vi "TimeCal.vi"(9 "Speed In":dbl format="%#_13g", 10 "Command":string, 11 "controller in":refnum<k24>) -> (2 "Time(ms)":dbl, 3 "controller out":refnum<k24>)   [LabVIEW 2016]
uses:
  C:/Users/TTUHEP/Documents/LabVIEW/Other Models/2010/Bin/Aerotech.A3200.dll
  Other Models/2010/Bin/Aerotech.A3200.dll
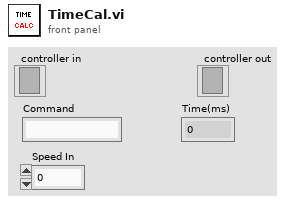
[diagram p1: front panel]
types:
  T1 = typedef "ControllerDiagPacket.ctl" = cluster{"Number of Diag Packets":i32, "Axes":T2[], "error":errorcluster}
  T2 = typedef "AxisDiagPacket.ctl" = cluster{"Axis Name":string, "Analog Input 0":dbl, "Analog Input 1":dbl, "Axis Fault (num)":i32, "Axis Fault (str)":string, "Axis Fault (bits)":cluster{"AmplifierFault":bool, "AmplifierTemperatureFault":bool, "CcwEndOfTravelLimitFault":bool, "CcwSoftwareLimitFault":bool, "CommunicationLostFault":bool, "CwEndOfTravelLimitFault":bool, "CwSoftwareLimitFault":bool, "EmergencyStopFault":bool, "EncoderFault":bool, "ExternalFault":bool, "FeedbackScalingFault":bool, "GantryMisalignFault ":bool, "HallSensorFault":bool, "InPositionTimeoutFault":bool, "InternalFault":bool, "MarkerSearchFault":bool, "MaxVelocityCommandFault":bool, "MissedInterruptFault":bool, "MotorTemperatureFault":bool, "None":bool, "OverCurrentFault":bool, "PositionErrorFault":bool, "PositionFeedbackFault":bool, "PowerSupplyFault":bool, "ProbeInputFault":bool, "SafeZoneFault":bool, "VelocityErrorFault":bool, "VelocityFeedbackFault":bool, "VoltageClampFault":bool}, "Axis Status (num)":i32, "Axis Status (str)":string, "Axis Status (bits)":cluster{"BacklashActive":bool, "CalibrationEnabled1D":bool, "CalibrationEnabled2D":bool, "CommandValid":bool, "DriveAbortPending":bool, "DrivePending":bool, "Enabling":bool, "GainMappingEnabled":bool, "GantryAligned":bool, "GantryRealigning":bool, "Homed":bool, "Homing":bool, "IFOVEnabled":bool, "JogGenerating":bool, "Jogging":bool, "JoystickControl":bool, "MasterSlaveControl":bool, "MotionBlocked":bool, "MotionClamped":bool, "MoveDone":bool, "None":bool, "NotVirtual":bool, "Profiling":bool, "Stability0":bool, "Stability1":bool, "TrajectoryFiltering":bool, "WaitDone":bool}, "Current Command":sgl, "Current Error":sgl, "Current Feedback":sgl, "Digital Inputs":i32, "Digital Outputs":i32, "Drive Status":i32, "Drive Status (str)":string, "Drive Status (bits)":cluster{"AccelerationPhase":bool, "AutofocusActive":bool, "BrakeOutput":bool, "CcwEndOfTravelLimitInput":bool, "CosineEncoderError":bool, "CurrentClamp":bool, "CwEndOfTravelLimitInput":bool, "DecelerationPhase":bool, "DualLoopActive":bool, "EmergencyStopInput":bool, "Enabled":bool, "EncoderClipping":bool, "GalvoCalibrationEnabled":bool, "GalvoPowerCorrection":bool, "HallAInput":bool, "HallBInput":bool, "HallCInput":bool, "HighResolutionMode":bool, "HomeLimitInput":bool, "InPosition":bool, "InPosition2":bool, "MarkerInput":bool, "MarkerLatch":bool, "MoveActive":bool, "NoMotorSupply":bool, "None":bool, "PowerLimiting":bool, "ProgrammingFlash":bool, "ProgrammingMXH":bool, "PSOHaltLatch":bool, "ServoControl":bool, "SineEncoderError":bool}, "Position Feedback Auxiliary":dbl, "Position Command":dbl, "Position Error":dbl, "Position Feedback":dbl, "Program Position Command":dbl, "Program Position Error":dbl, "Program Position Feedback":dbl, "Velocity Command":dbl, "Velocity Error":dbl, "Velocity Feedback":dbl}
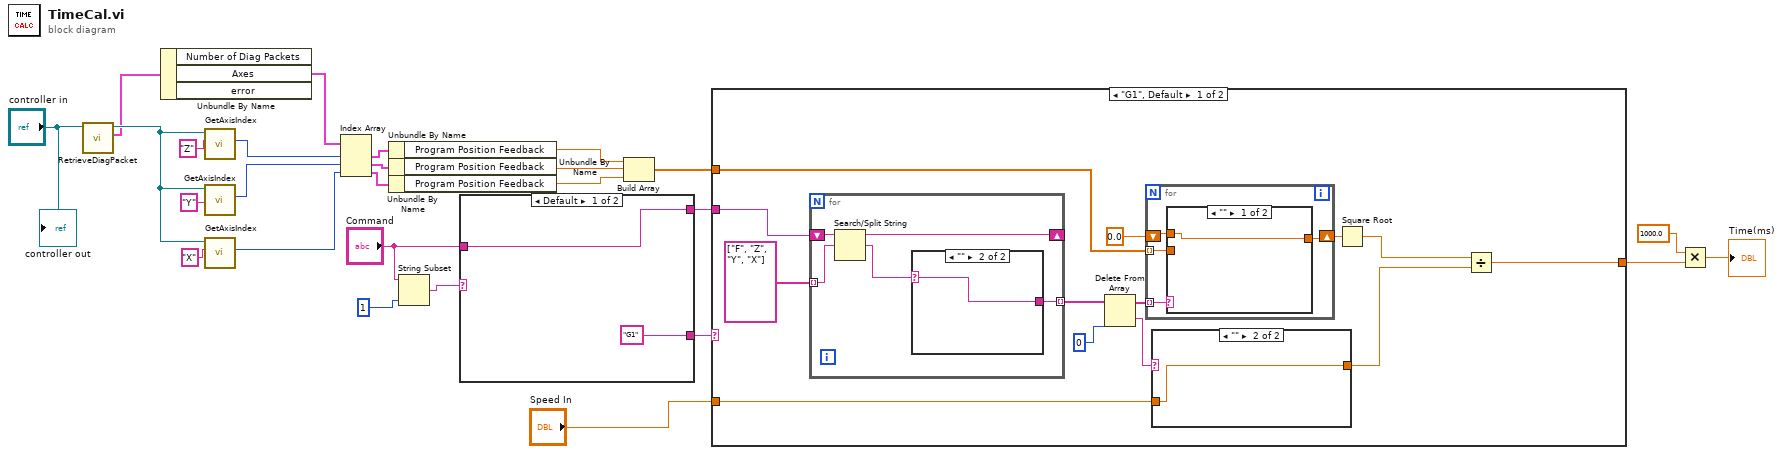
[diagram p0: block diagram]
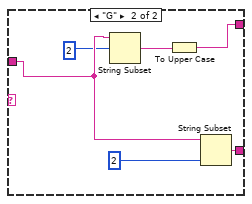
[diagram p2: hidden frame]
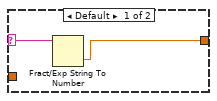
[diagram p3: hidden frame]
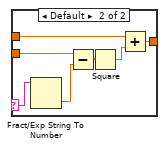
[diagram p4: hidden frame]
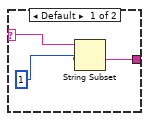
[diagram p5: hidden frame]
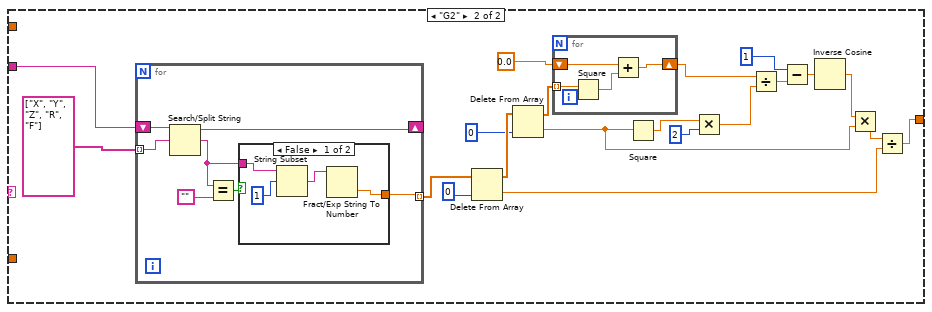
[diagram p6: hidden frame]
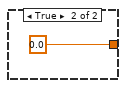
[diagram p7: hidden frame]
diagram:
  n1 = call "RetrieveDiagPacket.vi"("Controller In"="controller in") -> ("ControllerDiagPacket"=w16:T1, "Controller Out"=w20:refnum<k24>)  [unwired: 8 in, 1 out]
  n2 = Unbundle By Name(w16) -> ("Axes"=w15:T2[])  [unwired: 2 out]
  n3 = call "GetAxisIndex.vi"("axis name"="Z", "controller in"=w20) -> ("axis index"=w14:i32)  [unwired: 7 in, 2 out]
  n4 = call "GetAxisIndex.vi"("axis name"="Y", "controller in"=w20) -> ("axis index"=w13:i32)  [unwired: 7 in, 2 out]
  n5 = call "GetAxisIndex.vi"("axis name"="X", "controller in"=w20) -> ("axis index"=w12:i32)  [unwired: 7 in, 2 out]
  n6 = Index Array(array=w15, index #1=w14, index #2=w13, index #3=w12) -> (element #1=w11:T2, element #2=w10:T2, element #3=w9:T2)
  n7 = Unbundle By Name(w11) -> ("Program Position Feedback"=w8:dbl)
  n8 = Unbundle By Name(w10) -> ("Program Position Feedback"=w7:dbl)
  n9 = Unbundle By Name(w9) -> ("Program Position Feedback"=w6:dbl)
  n10 = String Subset(string="Command", length (rest)=1) -> (substring=w2:string)  [unwired: 1 in]
  n11 = case shown="Default" w2 {
    tunnel: ["G1" w34] -> w26
    tunnel: [w27 w33] -> w25
    tunnel: "Command" -> [w27 w30]
    frame Default {
    }
    frame "G" {
      n12 = String Subset(string=w30, offset (0)=2) -> (substring=w31:string)  [unwired: 1 in]
      n13 = To Upper Case(1:w31) -> (0:w33:string)
      n14 = String Subset(string=w30, length (rest)=2) -> (substring=w34:string)  [unwired: 1 in]
    }
  }
  n15 = Build Array(w8, w7, w6) -> (w5:dbl[])
  n16 = case shown="\"G1\", Default" w26 {
    tunnel: w25 -> [w46 w90]
    tunnel: [w39 w72] -> w24
    tunnel: w5 -> [w38 _]
    tunnel: "Speed In" -> [w36 _]
    frame "G1", Default {
      n17 = for {
        tunnel: string[] ["F", "Z", "Y", "X"] -> [w67] mode=indexing
        shift-right: [w65] -> _
        shift-left: w46 -> [w66]
        tunnel: [w64] -> w45 mode=indexing
        n18 = Search/Split String(string=w66, search string/char (-)=w67) -> (substring before match=w65:string, match + rest of string=w63:string)  [unwired: 1 in, 1 out]
        n19 = case shown="\"\"" w63 {
          selector: w63 -> [w68 w71]
          tunnel: [w69 w71] -> w64
          frame Default {
            n20 = String Subset(string=w68, offset (0)=1) -> (substring=w69:string)  [unwired: 1 in]
          }
          frame "" {
          }
        }
      }
      n21 = Delete From Array(array=w45, index=0) -> (deleted portion=w37:string, array with subset deleted=w43:string[])  [unwired: 1 in]
      n22 = for {
        tunnel: w43 -> [w53] mode=indexing
        shift-right: [w54] -> w41
        shift-left: 0.0 -> [w52]
        tunnel: w38 -> [w51] mode=indexing
        n23 = case shown="\"\"" w53 {
          selector: w53 -> [_ w57]
          tunnel: [w55 w61] -> w54
          tunnel: w52 -> [w55 w59]
          tunnel: w51 -> [_ w58]
          frame "" {
          }
          frame Default {
            n24 = Fract/Exp String To Number(string=w57) -> (number=w56:dbl)  [unwired: 3 in, 1 out]
            n25 = Subtract(x=w58, y=w56) -> (x-y=w60:dbl)
            n26 = Square(x=w60) -> (x^2=w62:dbl)
            n27 = Add(x=w59, y=w62) -> (x+y=w61:dbl)
          }
        }
      }
      n28 = case shown="\"\"" w37 {
        selector: w37 -> [w49 _]
        tunnel: w36 -> [_ w50]
        tunnel: [w48 w50] -> w35
        frame Default {
          n29 = Fract/Exp String To Number(string=w49) -> (number=w48:dbl)  [unwired: 3 in, 1 out]
        }
        frame "" {
        }
      }
      n30 = Square Root(x=w41) -> (sqrt(x)=w40:dbl)
      n31 = Divide(x=w40, y=w35) -> (x/y=w39:dbl)
    }
    frame "G2" {
      n32 = for {
        tunnel: string[] ["X", "Y", "Z", "R", "F"] -> [w101] mode=indexing
        shift-right: [w100] -> _
        shift-left: w90 -> [w102]
        tunnel: [w96] -> w89 mode=indexing
        n33 = Search/Split String(string=w102, search string/char (-)=w101) -> (substring before match=w100:string, match + rest of string=w97:string)  [unwired: 1 in, 1 out]
        n34 = Equal?(x=w97, y="") -> (x = y?=w99:bool)
        n35 = case shown="False" w99 {
          tunnel: w97 -> [w106 _]
          tunnel: [w104 0.0] -> w96
          frame False {
            n36 = String Subset(string=w106, offset (0)=1) -> (substring=w103:string)  [unwired: 1 in]
            n37 = Fract/Exp String To Number(string=w103) -> (number=w104:dbl)  [unwired: 3 in, 1 out]
          }
          frame True {
          }
        }
      }
      n38 = Delete From Array(array=w89, index=0) -> (deleted portion=w73:dbl, array with subset deleted=w87:dbl[])  [unwired: 1 in]
      n39 = Delete From Array(array=w87, index=0) -> (deleted portion=w76:dbl, array with subset deleted=w85:dbl[])  [unwired: 1 in]
      n40 = for {
        tunnel: w85 -> [w95] mode=indexing
        shift-right: [w94] -> w83
        shift-left: 0.0 -> [w93]
        n41 = Square(x=w95) -> (x^2=w92:dbl)
        n42 = Add(x=w93, y=w92) -> (x+y=w94:dbl)
      }
      n43 = Square(x=w76) -> (x^2=w82:dbl)
      n44 = Multiply(x=w82, y=2) -> (x*y=w80:dbl)
      n45 = Divide(x=w83, y=w80) -> (x/y=w79:dbl)
      n46 = Subtract(x=1, y=w79) -> (x-y=w77:dbl)
      n47 = Inverse Cosine(1:w77) -> (0:w75:dbl)
      n48 = Multiply(x=w75, y=w76) -> (x*y=w74:dbl)
      n49 = Divide(x=w74, y=w73) -> (x/y=w72:dbl)
    }
  }
  n50 = Multiply(x=1000.0, y=w24) -> (x*y=→"Time(ms)":dbl)
  "controller out" <- "controller in"
